vi "Read Default From File.vi"(8 "error in (no error)":errorcluster, 9 "Name":string, 10 "Path":path, 11 "Path Settings in":refnum<class "Path Settings.lvclass">) -> (0 "error out":errorcluster, 3 "Path Settings out":refnum<class "Path Settings.lvclass">)   [LabVIEW 2019, in "Path Settings.lvclass"]
uses:
  Path Settings.lvclass
  ObjectSettings/ObjectSettings.lvclass
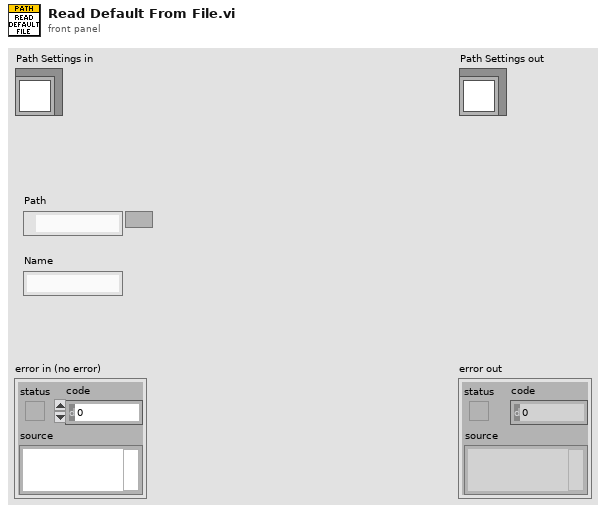
[diagram p1: front panel]
types:
  T1 = typedef "Path Settings.lvclass/Default Path Cluster.ctl" = cluster{"Fill Orientation":u16, "Smooth Segments":dbl, "Fill Spacing":dbl, "Interpolation":dbl}
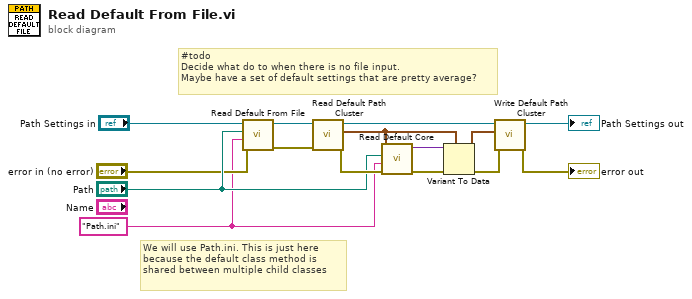
[diagram p0: block diagram]
diagram:
  w1 = "Path.ini"
  # "We will use Path.ini. This is just here because the default class method is shared between multiple child classes"
  # "#todo\nDecide what do to when there is no file input.\nMaybe have a set of default settings that are pretty average?"
  n1 = call-parent "Read Default From File.vi"("error in (no error)"="error in (no error)", "Name"=w1, "Path"="Path", "ObjectSettings in"="Path Settings in") -> ("error out"=w9:errorcluster, "ObjectSettings out"=w12:refnum<class "Path Settings.lvclass">)  [unwired: 6 in]
  n2 = call "Read Default Path Cluster.vi"("error in (no error)"=w9, "Path Settings in"=w12) -> ("error out"=w5:errorcluster, "Default Path"=w8:T1, "Path Settings out"=w11:refnum<class "Path Settings.lvclass">)  [unwired: 7 in]
  n3 = call "Read Default Core.vi"("error in (no error)"=w5, "Name"=w1, "Path"="Path", "Cluster In"=w8) -> ("error out"=w14:errorcluster, "Cluster Out"=w13:variant)  [unwired: 6 in]
  n4 = Variant To Data(error in=w14, type=w8, Variant=w13) -> (data=w7:T1, error out=w6:errorcluster)
  n5 = call "Write Default Path Cluster.vi"("error in (no error)"=w6, "Default Path"=w7, "Path Settings in"=w11) -> ("error out"=→"error out":errorcluster, "Path Settings out"=→"Path Settings out":refnum<class "Path Settings.lvclass">)  [unwired: 7 in]
